vi "NI 5772 (AC) - Digitizer_vDirectDataSend (FPGA) V3.vi"() -> ()   [LabVIEW 2020]
doc: "Example Description:\nThis example demonstrates how to enable Time Interleaved Sampling with the NI 5772 adapter module to achieve a sampling rate of 1.6GS/s. This example continuously acquires records of analog input data from the NI 5772 adapter module. It allows you to select an AI channel, trigger type, and record size. This VI must be compiled before it is run. \n\nRunning the VI:\nThis VI must be run from the NI 5772 - Getting Started (Host).vi. Refer to the host VI documentation for steps regarding running and configuring the FPGA VI. \n\nExecution Steps:\nRefer to the Block Diagram of this VI for execution comments."
uses:
  Controls/AI Trigger Type.ctl
  Controls/DigitizerState.ctl
  Controls/Aquire State.ctl
  <vilib>/Platform/TimedLoop/XDataNode/timing_clust.ctl
  <vilib>/Platform/TimedLoop/XDataNode/nitl_modes.ctl
  <vilib>/Platform/TimedLoop/XDataNode/wakeup.ctl
  <vilib>/rvi/Emulation/niFpgaGetClockAttributes.vi
  <vilib>/rvi/Emulation/niFpgaSctlEmulationGetInTimedLoop.vi
  <vilib>/rvi/Emulation/niFpgaEmulationReportErrorSimple.vi
  <vilib>/rvi/eio/common/nirviEmuTemplateMethod_errors.vi
  <vilib>/rvi/Emulation/niFpgaCriticalErrorInLSC.vi
  <vilib>/rvi/Emulation/niFpgaProcessEmulError.vi
  <vilib>/rvi/Emulation/niFpgaEmulationIsFPGAContextNoSignature.vi
  <vilib>/rvi/errors/niFpgaSetErrorForExecOnDevCompSimple.vi
  <vilib>/rvi/eio/common/nirviEmuReportErrorAndStop.vi
  <vilib>/rvi/DataTransferAndStorage/Container/Common/niFpgaContainerGetUniqueNameForEmu.vi
  <vilib>/rvi/FIFO/Fifo_Resource/nirvififoEmulationSetSize.vi
  <vilib>/rvi/FIFO/Fifo_Resource/nirviFifoEmulationQueueMgr.vi
  <instcachedir>/0/nirviFifoEmulationQueueMgr_E5CAEC123FF24DC58D834DCA3CDAA9B5.lvgen/nirviFifoEmulationQueueMgr_E5CAEC123FF24DC58D834DCA3CDAA9B5_004.vi
  <vilib>/Utility/error.llb/Clear Errors.vi
  <vilib>/rvi/FIFO/Fifo_Resource/nirvififoEmulationCreateLock.vi
  <vilib>/rvi/FIFO/Fifo_Resource/nirvififoEmulationObtainLock.vi
  <vilib>/rvi/FIFO/Fifo_Resource/nirvififoEmulationReleaseLock.vi
  <vilib>/rvi/occurrence/nirviWaitOnOccurrenceBase.vi
  <vilib>/rvi/errors/nirviReportUnexpectedCaseInternalError.vi
  <vilib>/rvi/errors/nirviReportUnexpectedCaseInternalError (U32).vi
  <vilib>/rvi/FIFO/Fifo_Resource/nirvififoEmulationDetermineInputValidOut.vi
  <instcachedir>/0/nirviFifoEmulationQueueMgr_E5CAEC123FF24DC58D834DCA3CDAA9B5.lvgen/nirviFifoEmulationQueueMgr_E5CAEC123FF24DC58D834DCA3CDAA9B5_000.vi
  <instrlib>/_niInstr/Basic Elements/v1/FPGA/Private/Count Up U64.vi
  <instcachedir>/0/nirviFifoEmulationQueueMgr_E5CAEC123FF24DC58D834DCA3CDAA9B5.lvgen/nirviFifoEmulationQueueMgr_E5CAEC123FF24DC58D834DCA3CDAA9B5_003.vi
  <vilib>/rvi/interface/RandomDataEmulation/niFpgaRandomDataHandleErrors.vi
  <vilib>/eio/EIONode/EIONode.xnode
  <vilib>/rvi/DataTransferAndStorage/Container/XNode/niFpgaContainer.xnode
  <vilib>/rvi/FIFO/Fifo_Resource/nirvififoEmulationRead.vi
  <vilib>/Platform/TimedLoop/XDataNode/XDataNode.xnode
  <vilib>/rvi/FIFO/Fifo_Resource/nirvififoEmulationWrite.vi
  <vilib>/rvi/FIFO/Fifo_Resource/nirvififoEmulationGetNumberOfElementsToRead.vi
  <vilib>/rvi/interface/RandomDataEmulation/nirviRandomDataFpgaReadWriteTemplate.vi
  <vilib>/Platform/TimedLoop/XDataNode/XDNodeRunTimeDep.lvlib
  <instrlib>/_niInstr/Basic Elements/v1/FPGA/niInstr Basic Elements v1 FPGA.lvlib
  <vilib>/rvi/Memory/Memory_Emulation/nirvimemoryFastEmulation.vi
  <vilib>/rvi/Memory/Memory_Emulation/nirvimemoryEmulation.vi
panel:
  out "Accumulator Length":u32
  out "Aquire Loop":T1
  out "Data Transfer Loop":T2
  out "DMA FIFO Overflow? 3":bool caption="FIFO Overflow?"
  out "DMA FIFO Overflow? 2":bool caption="FIFO Overflow?"
  out "WaitForWave\nCompletion":u16
  in  "Wave Sampling Rate":sgl
  in  "WaveSampleCount":sgl format="%#_13g"
  in  "Delay (us)":sgl
  in  "AvgCount_powerOf2":i16=1
  out "DMA FIFO Overflow?":bool caption="FIFO Overflow?"
  out "Removed\nElement":u64
  out "AvgCount":u16=1
  in  "vi/nGenTrig":bool
  in  "TrigIn Simulate":bool
  out "Trig Count":u64
  in  "Clear Count":bool
  out "Delay after Trig [cycles]":u16
  out "TS FIFO In Overflow?":bool caption="FIFO Overflow?"
  in  "Samples Per Trigger":u16=512 min=1 step=1
  in  "Arm Trigger":bool
  in  "User Command Commit":bool
  in  "User Command":u8
  out "User Command Idle":bool
  out "User Command Status":u8
  in  "User Data 0":u16
  in  "User Data 1":u8
  out "PLL Locked":bool
  out "User Error":bool
  out "Configured?":bool
  in  "Trigger Level":i16
  in  "Trigger Type":T3
  # "Resource Configuration"
  # "Analog Input"
  # "Clock Configuration"
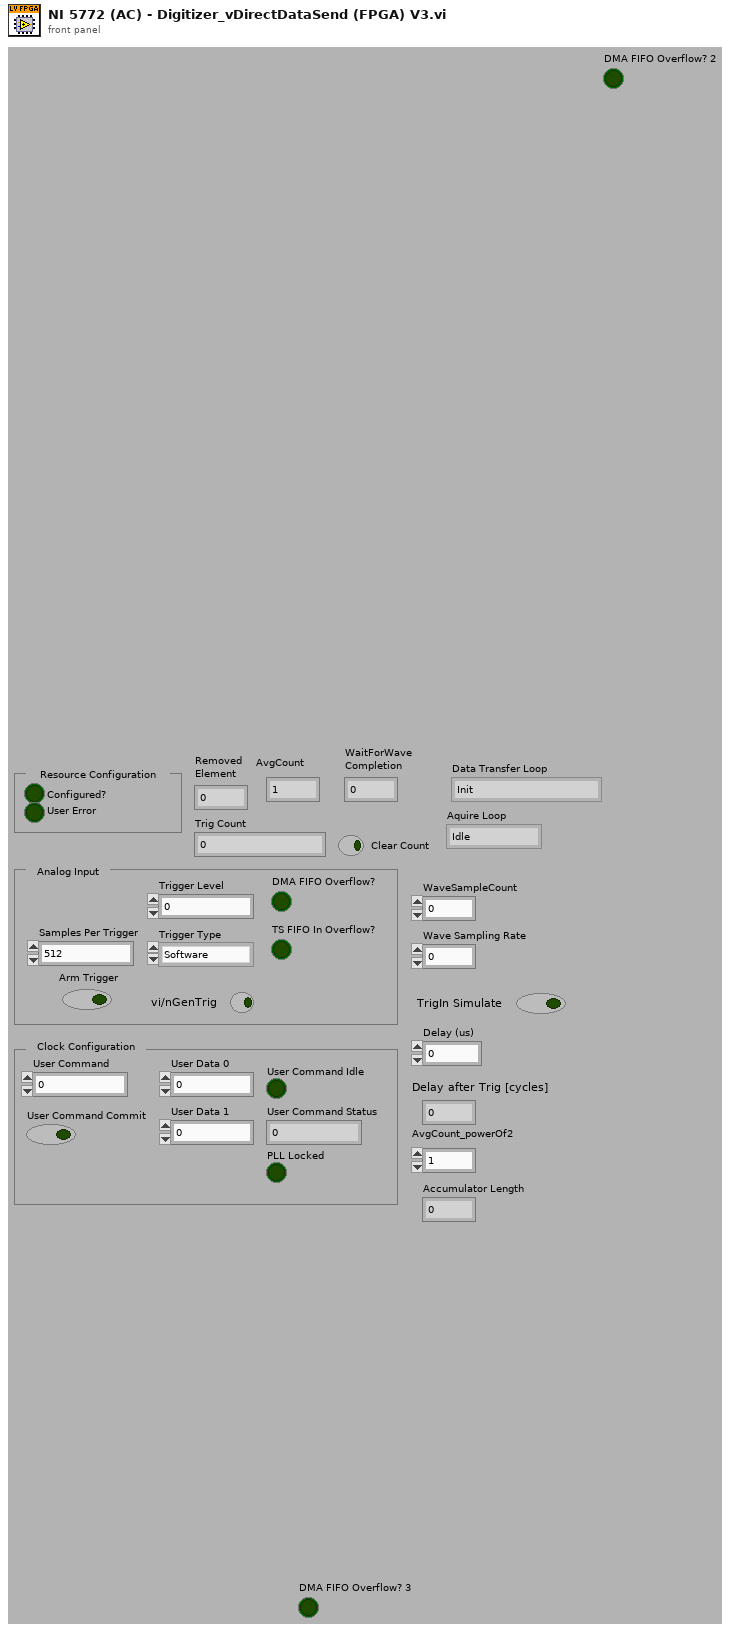
[diagram p1: front panel]
types:
  T1 = typedef "Aquire State.ctl" = enum8{"Idle", "Wait for Trigger", "AlignWave", "Hold Aquire", "Acquire", "WaitForWaveCompletion", "CheckAvg"}
  T2 = typedef "DigitizerState.ctl" = enum16{"Init", "Build/Clear Accumulator", "GetData", "AverageCountCheck", "SendtoHost"}
  T3 = typedef "AI Trigger Type.ctl" = enum8{"Software", "Data Edge"}
  T4 = typedef "XDNodeRunTimeDep.lvlib/timing_clust.ctl" = cluster{"Expected End [f-1]":u64, "Actual End [f-1]":u64, "Finished Late? [f-1]":bool, "Expected End [i-1]":u64, "Actual End [i-1]":u64, "Finished Late? [i-1]":bool, "Expected Start [i]":u64, "Actual Start [i]":u64, "Expected Start [f]":u64, "Actual Start [f]":u64, "Source Name":string, "Structure Name":string, "Period":i64, "Deadline":i64, "Offset":i64, "Start":i64, "Priority":i32, "Timeout":i32, "Mode":T5, "Wakeup Reason":T6, "Error":errorcluster, "Source Type":string, "Secondary Source Type":string, "Global End Time":u64, "Global Start Time":u64, "Frame Duration":u64, "Iteration Duration":u64, "Assigned CPU":i32, "I/O Scan Engine Mode":u32}
  T5 = typedef "XDNodeRunTimeDep.lvlib/nitl_modes.ctl" = enum32{"No Change", "Process missed periods, maintain original phase", "Discard missed periods, maintain original phase", "Process missed periods, ignore original phase", "Discard missed periods, ignore original phase"}
  T6 = typedef "XDNodeRunTimeDep.lvlib/wakeup.ctl" = enum32{"Normal", "Aborted", "Asynchronous wakeup", "Timing source error", "Timed loop error", "Timeout"}
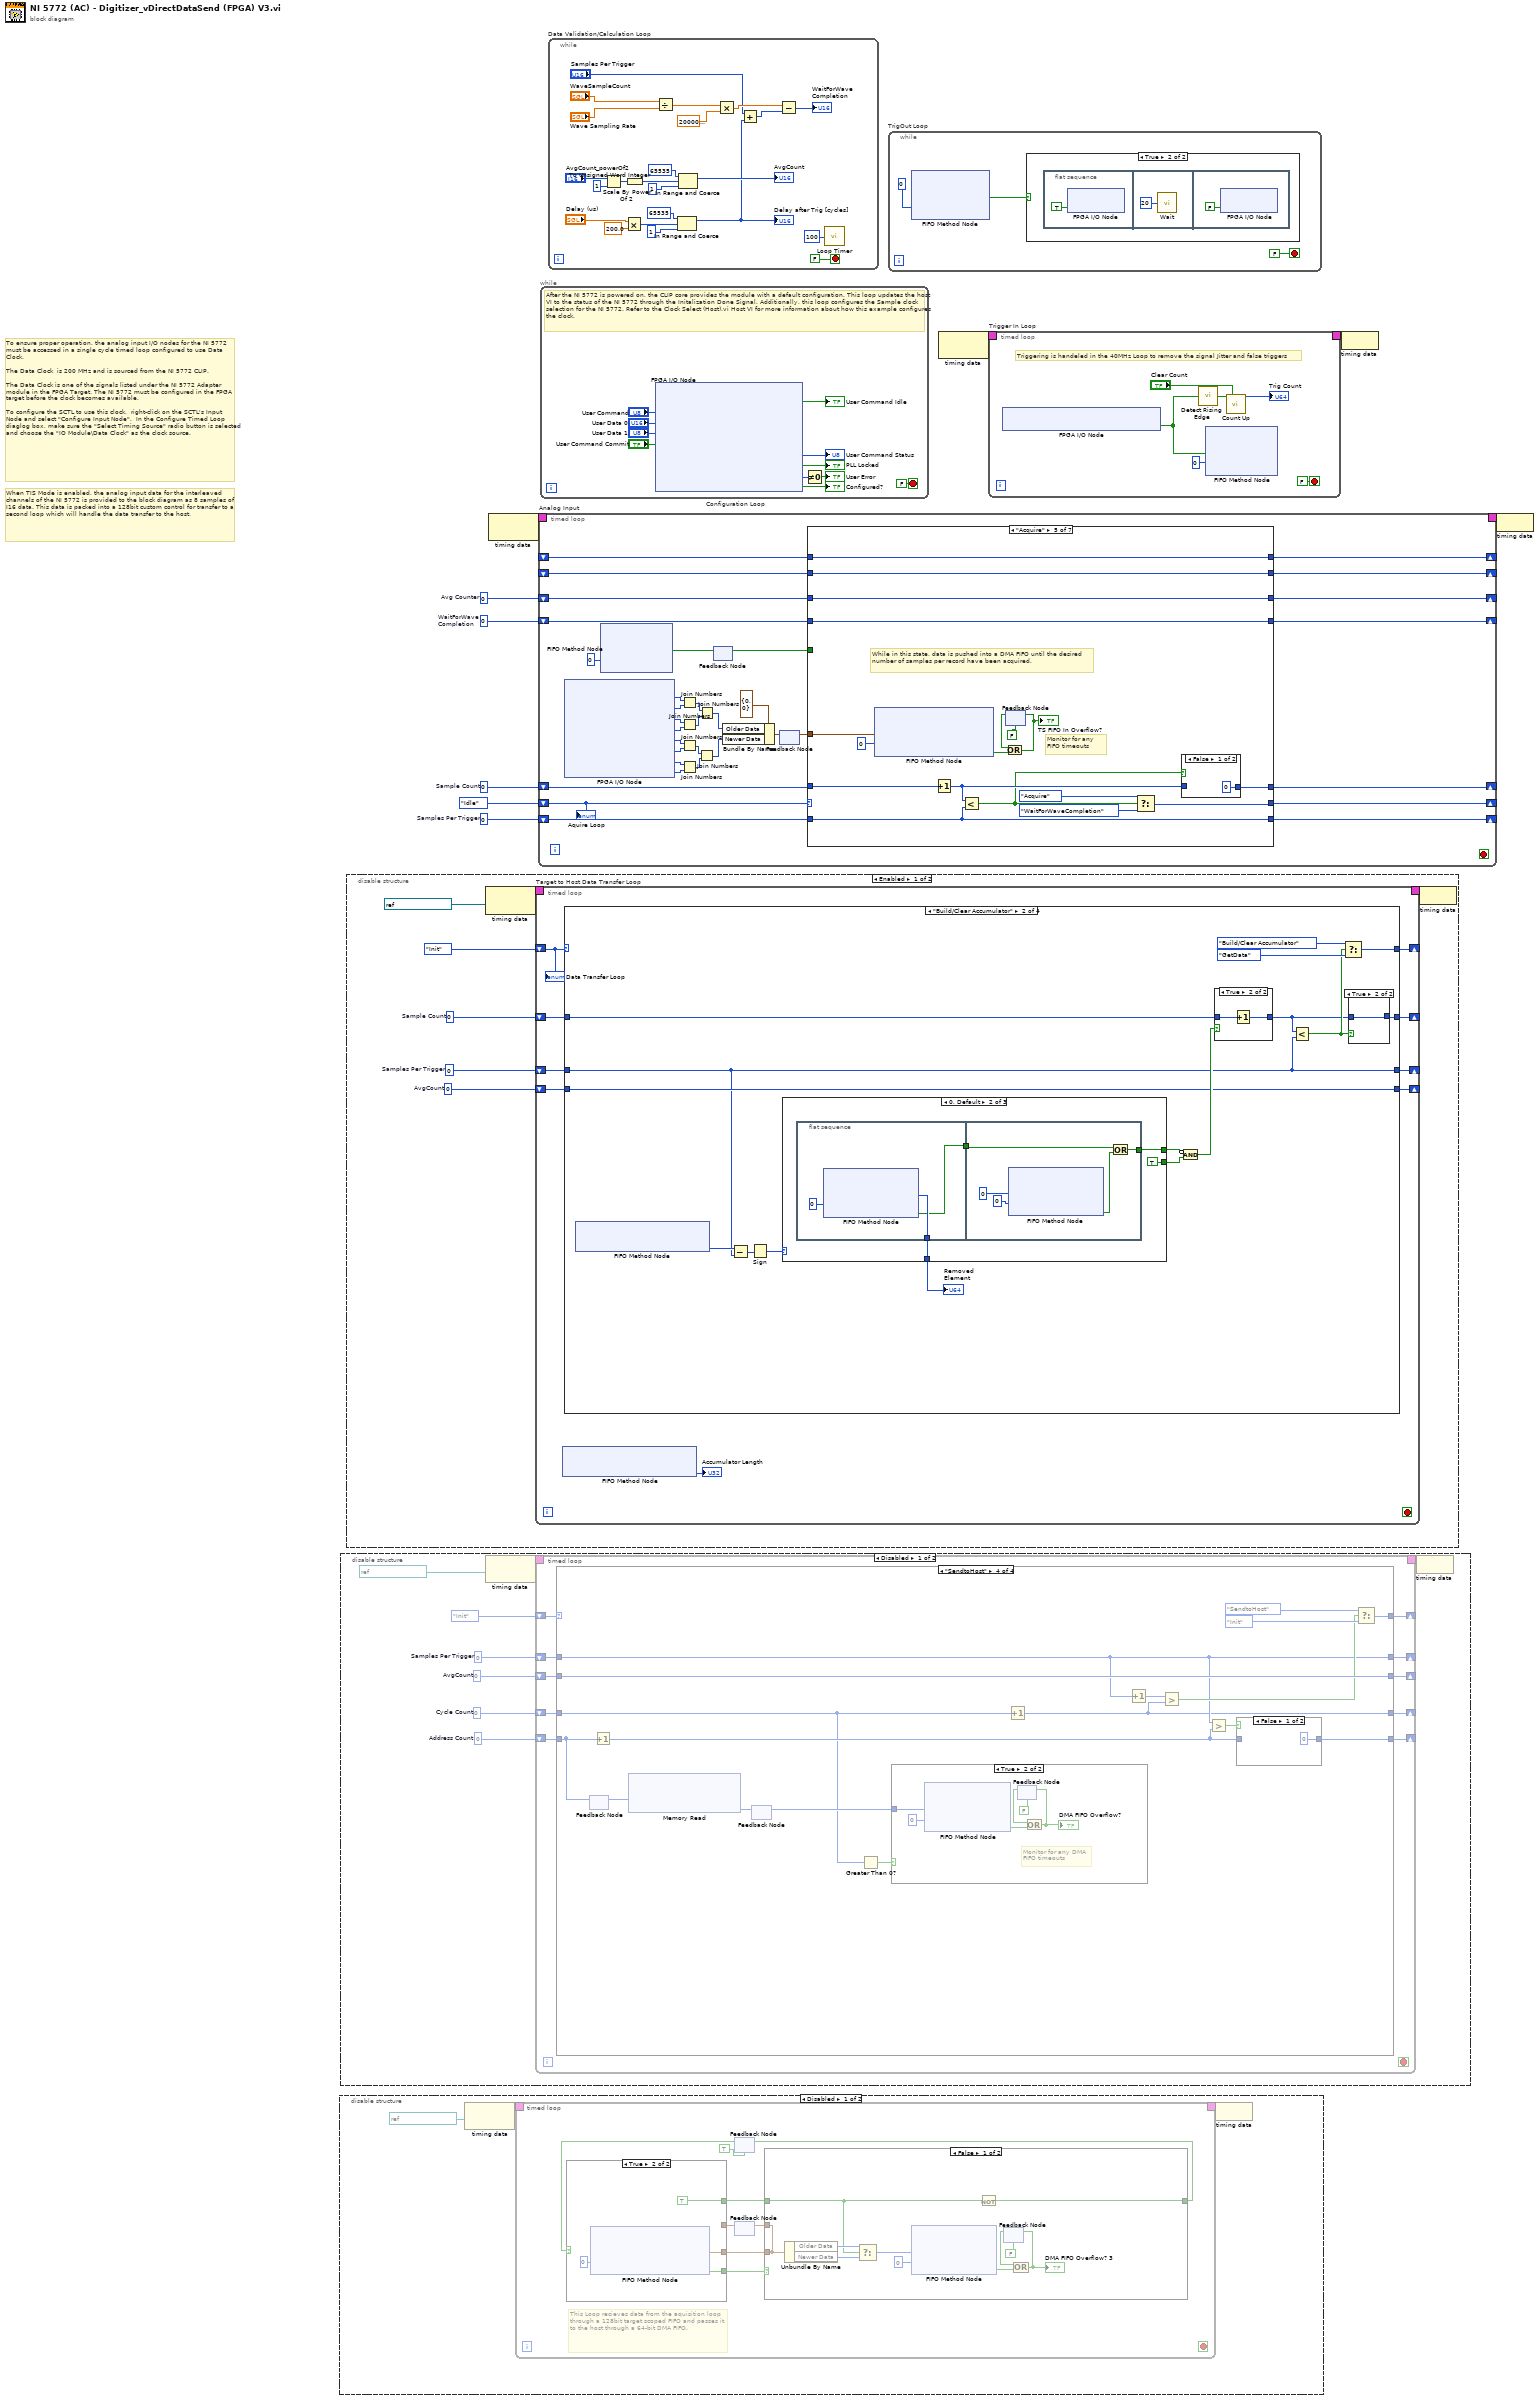
[diagram p0: block diagram]
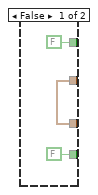
[diagram p2: hidden frame]
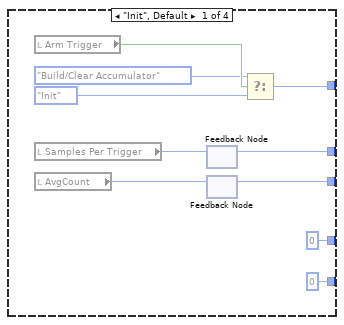
[diagram p5: hidden frame]
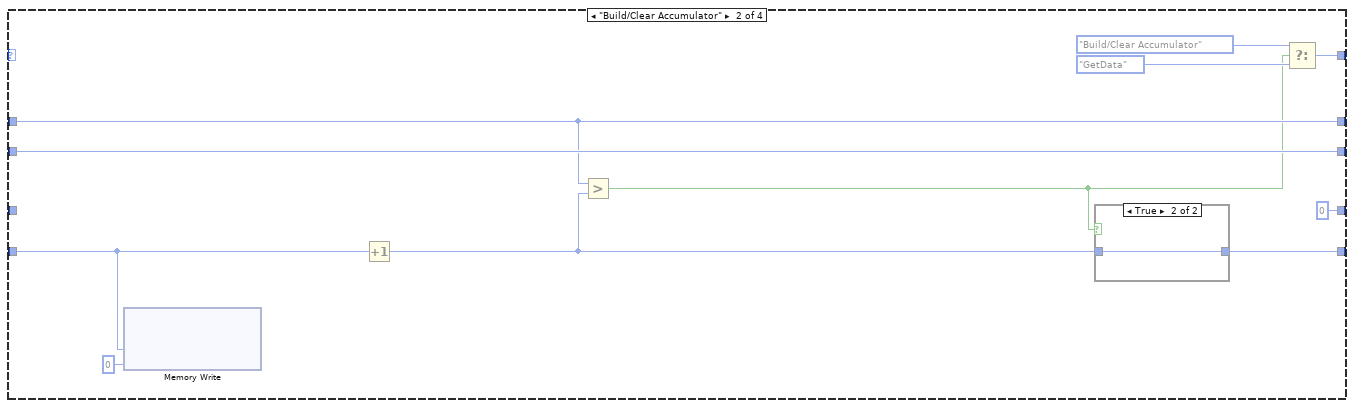
[diagram p6: hidden frame]
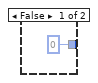
[diagram p7: hidden frame]
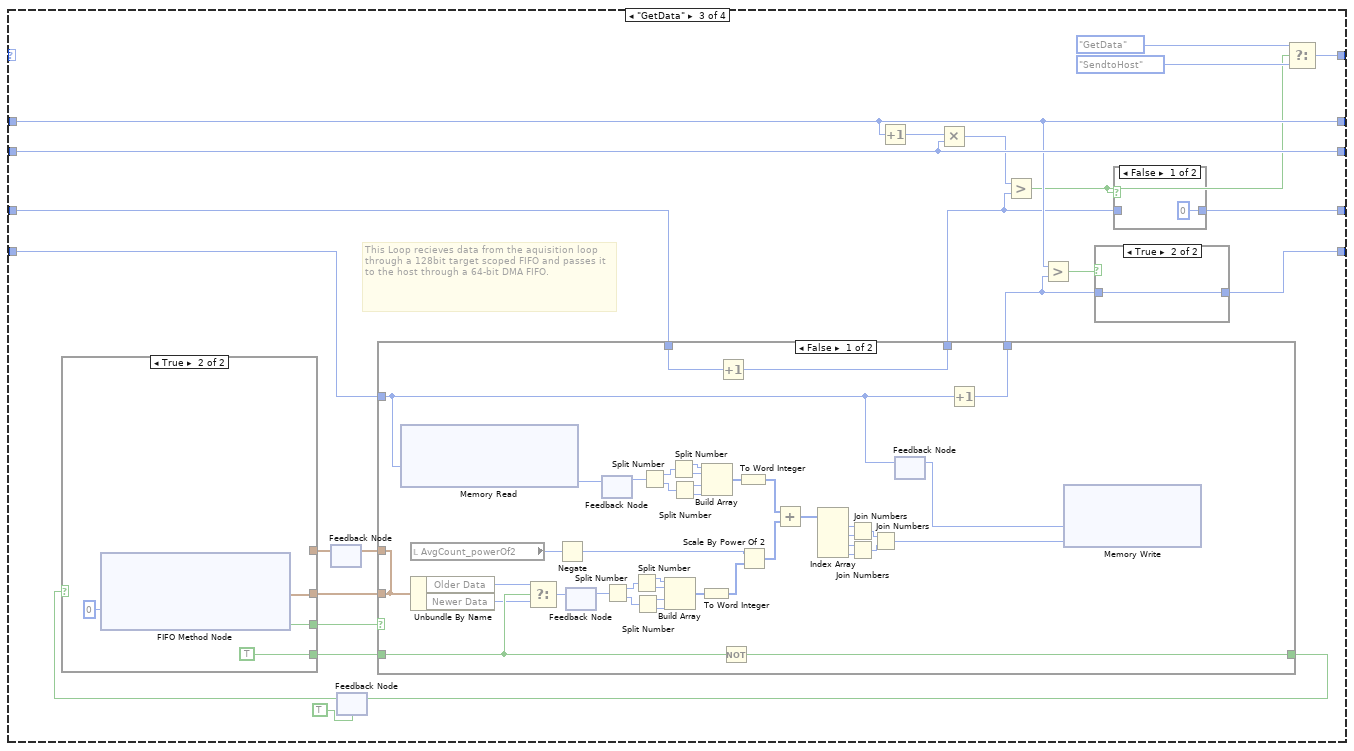
[diagram p8: hidden frame]
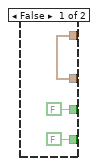
[diagram p10: hidden frame]
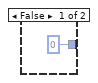
[diagram p12: hidden frame]
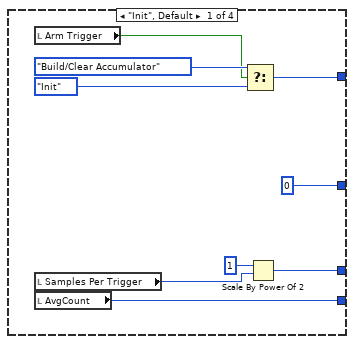
[diagram p16: hidden frame]
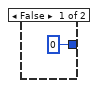
[diagram p17: hidden frame]
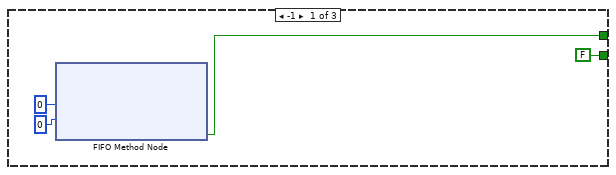
[diagram p19: hidden frame]
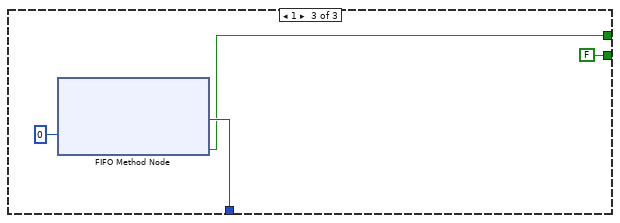
[diagram p20: hidden frame]
diagram:
  w1 = u16 0  # WaitForWave Completion
  w2 = u16 0  # Avg Counter
  w5 = u16 0  # Samples Per Trigger
  w6 = u16 0  # Sample Count
  # "When TIS Mode is enabled, the analog input data for the interleaved channels of the NI 5772 is provided to the block diagram as 8 samples of I16 data. This data is packed into a 128bit custom control for transfer to a second loop which will handle the data transfer to the host."
  # "To ensure proper operation, the analog input I/O nodes for the NI 5772 must be accessed in a single cycle timed loop configured to use Data Clock. \n\nThe Data Clock  is 200 MHz and is sourced from the NI 5772 CLIP.\n\nThe Data Clock is one of the signals listed under the NI 5772 Adapter module in the FPGA Target. The NI 5772 must be configured in the FPGA target before the clock becomes available. \n\nTo configure the SCTL to use this clock,  right-click on the SCTL's Input Node and select \"Configure Input Node\".  In the Configure Timed Loop diaglog box, make sure the \"Select Timing Source\" radio button is selected and choose the \"IO Module\\Data Clock\" as the clock source."
  n1 = disable-structure shown="Disabled" {
    frame Disabled {
      n2 = node-c288(refnum<k21> "100 MHz Clock" ("Source Name")) -> (w12:T4)
      n3 = timed-loop {
        timing: w12 -> [_]
        timing-out: [_] -> w11
        stop <- _ stop-if-true
        # "This Loop recieves data from the aquisition loop through a 128bit target scoped FIFO and passes it to the host through a 64-bit DMA FIFO."
        n4 = feedback #1(TRUE ("Timed Out?")) -> (w15:bool)
        n5 = feedback #2() -> (w16:cluster{"Older Data":u64, "Newer Data":u64})  [unwired: 1 in]
        n6 = case shown="True" w15 {
          tunnel: [w21 w24] -> w18
          tunnel: [FALSE ("Timed Out?") w25] -> w20
          tunnel: [FALSE ("Timed Out?") TRUE ("Timed Out?")] -> w19
          tunnel: w16 -> [w21 _]
          frame False {
          }
          frame True {
            n7 = xnode ("FIFO Method Node")("Timeout"=0) -> ("Element"=w24:cluster{"Older Data":u64, "Newer Data":u64}, "Timed Out?"=w25:bool)  [unwired: 1 in, 1 out]
          }
        }
        n8 = case shown="False" w20 {
          tunnel: [w36 w40] -> w14
          tunnel: w19 -> [w37 w40]
          tunnel: w18 -> [w35 w39]
          tunnel: [w35 w39] -> w17
          frame False {
            n9 = Unbundle By Name(w35) -> ("Older Data"=w38:u64, "Newer Data"=w34:u64)
            n10 = Select(t=w38, s=w37, f=w34) -> (s? t:f=w28:u64)
            n11 = xnode ("FIFO Method Node")("Element"=w28, "Timeout"=0) -> ("Timed Out?"=w30:bool)  [unwired: 1 in, 1 out]
            n12 = Not(x=w37) -> (.not. x?=w36:bool)
            n13 = feedback #3(FALSE) -> (w31:bool)
            n14 = Compound Arithmetic op=OR(w31, w30) -> (w29:bool)
            "DMA FIFO Overflow? 3" <- w29
            n15 = feedback-in #3(w29) -> ()
          }
          frame True {
          }
        }
        n16 = feedback-in #1(w14) -> ()
        n17 = feedback-in #2(w17) -> ()
      }
      n18 = node-c288(w11) -> ()
    }
    frame Enabled {
    }
  }
  n19 = disable-structure shown="Disabled" {
    frame Disabled {
      w47 = u32 0  # Cycle Count
      w48 = u32 0  # Address Count
      w49 = u16 0  # AvgCount
      w50 = u16 0  # Samples Per Trigger
      n20 = node-c288(refnum<k21> "100 MHz Clock" ("Source Name")) -> (w54:T4)
      n21 = timed-loop {
        timing: w54 -> [_]
        timing-out: [_] -> w53
        shift-right: [w63] -> _
        shift-left: DigitizerState."Init" -> [w64]
        shift-right: [w62] -> _
        shift-left: w50 -> [w60]
        shift-right: [w61] -> _
        shift-left: w49 -> [w59]
        shift-right: [w57] -> _
        shift-left: w48 -> [w58]
        shift-right: [w55] -> _
        shift-left: w47 -> [w56]
        stop <- _ stop-if-true
        n22 = case shown="\"SendtoHost\"" w64 {
          tunnel: [w69 w79 w108 w180] -> w63
          tunnel: [w68 w82 w92 w170] -> w62
          tunnel: [w67 w83 w98 w183] -> w61
          tunnel: w60 -> [_ w82 w92 w170]
          tunnel: w59 -> [_ w83 w98 w183]
          tunnel: w58 -> [_ w85 w95 w172]
          tunnel: [u32 0 w76 w107 w178] -> w57
          tunnel: w56 -> [_ _ w91 w167]
          tunnel: [u32 0 ("Cycle Count") u32 0 ("Cycle Count") w88 w168] -> w55
          frame "Init", Default {
            n23 = local read "Arm Trigger"() -> (w74:bool)
            n24 = local read "Samples Per Trigger"() -> (w70:u16)
            n25 = local read "AvgCount"() -> (w71:u16)
            n26 = feedback #4() -> (w68:u16)  [unwired: 1 in]
            n27 = feedback-in #4(w70) -> ()
            n28 = feedback #5() -> (w67:u16)  [unwired: 1 in]
            n29 = feedback-in #5(w71) -> ()
            n30 = Select(t=DigitizerState."Build/Clear Accumulator", s=w74, f=DigitizerState."Init") -> (s? t:f=w69:T2)
          }
          frame "Build/Clear Accumulator" {
            n31 = xnode ("Memory Write")("Address"=w85, "Data"=u64 0) -> ()  [unwired: 1 in, 1 out]
            n32 = Increment(x=w85) -> (x+1=w77:u32)
            n33 = Greater?(x=w82, y=w77) -> (0:w78:bool)
            n34 = case shown="True" w78 {
              tunnel: w77 -> [_ w87]
              tunnel: [u32 0 w87] -> w76
              frame False {
              }
              frame True {
              }
            }
            n35 = Select(t=DigitizerState."Build/Clear Accumulator", s=w78, f=DigitizerState."GetData") -> (s? t:f=w79:T2)
          }
          frame "GetData" {
            # "This Loop recieves data from the aquisition loop through a 128bit target scoped FIFO and passes it to the host through a 64-bit DMA FIFO."
            n36 = feedback #6() -> (w102:cluster{"Older Data":u64, "Newer Data":u64})  [unwired: 1 in]
            n37 = feedback #7(TRUE ("Timed Out?")) -> (w101:bool)
            n38 = case shown="True" w101 {
              tunnel: [w113 w116] -> w104
              tunnel: [FALSE ("Timed Out?") w117] -> w106
              tunnel: [FALSE ("Timed Out?") TRUE ("Timed Out?")] -> w105
              tunnel: w102 -> [w113 _]
              frame False {
              }
              frame True {
                n39 = xnode ("FIFO Method Node")("Timeout"=0) -> ("Element"=w116:cluster{"Older Data":u64, "Newer Data":u64}, "Timed Out?"=w117:bool)  [unwired: 1 in, 1 out]
              }
            }
            n40 = case shown="False" w106 {
              tunnel: [w158 w164] -> w100
              tunnel: w105 -> [w159 w164]
              tunnel: w104 -> [w157 w163]
              tunnel: [w157 w163] -> w103
              tunnel: w95 -> [w134 w162]
              tunnel: [w147 w162] -> w94
              tunnel: w91 -> [w123 w161]
              tunnel: [w122 w161] -> w89
              frame False {
                n41 = xnode ("Memory Read")("Address"=w134) -> ("Data"=w125:u64)  [unwired: 1 in, 1 out]
                n42 = local read "AvgCount_powerOf2"() -> (w138:i16)
                n43 = Unbundle By Name(w157) -> ("Older Data"=w160:u64, "Newer Data"=w156:u64)
                n44 = Select(t=w160, s=w159, f=w156) -> (s? t:f=w148:u64)
                n45 = Negate(x=w138) -> (-x=w139:i16)
                n46 = feedback-in #8(w148) -> ()
                n47 = feedback #8() -> (w121:u64)  [unwired: 1 in]
                n48 = feedback-in #9(w125) -> ()
                n49 = feedback #9() -> (w124:u64)  [unwired: 1 in]
                n50 = Split Number(x=w121) -> (hi(x)=w150:u32, lo(x)=w151:u32)
                n51 = Split Number(x=w150) -> (hi(x)=w152:u16, lo(x)=w153:u16)
                n52 = Split Number(x=w151) -> (hi(x)=w154:u16, lo(x)=w155:u16)
                n53 = Split Number(x=w124) -> (hi(x)=w146:u32, lo(x)=w145:u32)
                n54 = Build Array(w152, w153, w154, w155) -> (w149:u16[])
                n55 = Split Number(x=w146) -> (hi(x)=w144:u16, lo(x)=w143:u16)
                n56 = Split Number(x=w145) -> (hi(x)=w142:u16, lo(x)=w141:u16)
                n57 = To Word Integer(number=w149) -> (16bit integer=w137:i16[])
                n58 = Build Array(w144, w143, w142, w141) -> (w140:u16[])
                n59 = Increment(x=w123) -> (x+1=w122:u32)
                n60 = Not(x=w159) -> (.not. x?=w158:bool)
                n61 = To Word Integer(number=w140) -> (16bit integer=w135:i16[])
                n62 = Scale By Power Of 2(n=w139, x=w137) -> (x*2^n=w136:i16[])
                n63 = Add(x=w135, y=w136) -> (x+y=w127:i16[])
                n64 = Index Array(array=w127) -> (element #1=w130:i16, element #2=w131:i16, element #3=w132:i16, element #4=w133:i16)  [unwired: 4 in]
                n65 = Join Numbers(hi=w130, lo=w131) -> ((hi.lo)=w128:u32)
                n66 = Join Numbers(hi=w132, lo=w133) -> ((hi.lo)=w129:u32)
                n67 = Join Numbers(hi=w128, lo=w129) -> ((hi.lo)=w126:u64)
                n68 = feedback-in #10(w134) -> ()
                n69 = feedback #10() -> (w120:u32)  [unwired: 1 in]
                n70 = Increment(x=w134) -> (x+1=w147:u32)
                n71 = xnode ("Memory Write")("Address"=w120, "Data"=w126) -> ()  [unwired: 1 in, 1 out]
              }
              frame True {
              }
            }
            n72 = feedback-in #6(w103) -> ()
            n73 = feedback-in #7(w100) -> ()
            n74 = Increment(x=w92) -> (x+1=w93:u16)
            n75 = Multiply(x=w93, y=w98) -> (x*y=w97:u16)
            n76 = Greater?(x=w97, y=w89) -> (0:w90:bool)
            n77 = Greater?(x=w92, y=w94) -> (0:w96:bool)
            n78 = case shown="True" w96 {
              tunnel: w94 -> [_ w166]
              tunnel: [u32 0 w166] -> w107
              frame False {
              }
              frame True {
              }
            }
            n79 = case shown="False" w90 {
              tunnel: w89 -> [_ w112]
              tunnel: [u32 0 ("Cycle Count") w112] -> w88
              frame False {
              }
              frame True {
              }
            }
            n80 = Select(t=DigitizerState."GetData", s=w90, f=DigitizerState."SendtoHost") -> (s? t:f=w108:T2)
          }
          frame "SendtoHost" {
            n81 = feedback-in #11(w172) -> ()
            n82 = feedback #11() -> (w174:u32)  [unwired: 1 in]
            n83 = Increment(x=w172) -> (x+1=w169:u32)
            n84 = xnode ("Memory Read")("Address"=w174) -> ("Data"=w177:u64)  [unwired: 1 in, 1 out]
            n85 = feedback-in #12(w177) -> ()
            n86 = feedback #12() -> (w176:u64)  [unwired: 1 in]
            n87 = Greater Than 0?(x=w167) -> (x > 0?=w173:bool)
            n88 = case shown="True" w173 {
              tunnel: w176 -> [_ w184]
              frame False {
              }
              frame True {
                # "Monitor for any DMA FIFO timeouts"
                n89 = xnode ("FIFO Method Node")("Element"=w184, "Timeout"=0) -> ("Timed Out?"=w188:bool)  [unwired: 1 in, 1 out]
                n90 = feedback #13(FALSE) -> (w187:bool)
                n91 = Compound Arithmetic op=OR(w187, w188) -> (w189:bool)
                "DMA FIFO Overflow?" <- w189
                n92 = feedback-in #13(w189) -> ()
              }
            }
            n93 = Increment(x=w167) -> (x+1=w168:u32)
            n94 = Increment(x=w170) -> (x+1=w175:u16)
            n95 = Greater?(x=w175, y=w168) -> (0:w179:bool)
            n96 = Greater?(x=w170, y=w169) -> (0:w171:bool)
            n97 = case shown="False" w171 {
              tunnel: w169 -> [_ w191]
              tunnel: [u32 0 w191] -> w178
              frame False {
              }
              frame True {
              }
            }
            n98 = Select(t=DigitizerState."SendtoHost", s=w179, f=DigitizerState."Init") -> (s? t:f=w180:T2)
          }
        }
      }
      n99 = node-c288(w53) -> ()
    }
    frame Enabled {
    }
  }
  n100 = disable-structure shown="Enabled" {
    frame Enabled {
      w198 = u16 0  # Sample Count
      w199 = u16 0  # Samples Per Trigger
      w200 = u16 0  # AvgCount
      n101 = node-c288(refnum<k21> "100 MHz Clock" ("Source Name")) -> (w204:T4)
      n102 = timed-loop "Target to Host Data Transfer Loop" {
        timing: w204 -> [_]
        timing-out: [_] -> w203
        shift-right: [w208] -> _
        shift-left: DigitizerState."Init" -> [w213]
        shift-right: [w212] -> _
        shift-left: w199 -> [w211]
        shift-right: [w210] -> _
        shift-left: w200 -> [w209]
        shift-right: [w206] -> _
        shift-left: w198 -> [w207]
        stop <- _ stop-if-true
        n103 = xnode ("FIFO Method Node")() -> ("Number of Elements to Read"=→"Accumulator Length":u32)  [unwired: 1 in, 1 out]
        n104 = case shown="\"Build/Clear Accumulator\"" w213 {
          tunnel: [w215 w226 w274 w348] -> w212
          tunnel: w211 -> [_ w226 w274 w348]
          tunnel: [w222 w227 w273 w355] -> w210
          tunnel: w209 -> [_ w227 w273 w355]
          tunnel: [w218 w234 w268 w351] -> w208
          tunnel: w207 -> [_ w229 w267 w349]
          tunnel: [u16 0 ("Sample Count") w223 w266 w346] -> w206
          frame "Init", Default {
            n105 = local read "Arm Trigger"() -> (w219:bool)
            n106 = local read "Samples Per Trigger"() -> (w214:u16)
            n107 = local read "AvgCount"() -> (w222:u16)
            n108 = Select(t=DigitizerState."Build/Clear Accumulator", s=w219, f=DigitizerState."Init") -> (s? t:f=w218:T2)
            n109 = Scale By Power Of 2(n=i16 1, x=w214) -> (x*2^n=w215:u16)
          }
          frame "Build/Clear Accumulator" {
            n110 = xnode ("FIFO Method Node")() -> ("Number of Elements to Read"=w238:u32)  [unwired: 1 in, 1 out]
            n111 = Subtract(x=w238, y=w226) -> (x-y=w237:i8)
            n112 = Sign(1:w237) -> (0:w236:i8)
            n113 = case shown="0, Default" w236 {
              tunnel: [_ w251 w262] -> w235
              tunnel: [w245 w249 w261] -> w231
              tunnel: [FALSE TRUE FALSE] -> w230
              frame -1 {
                n114 = xnode ("FIFO Method Node")("Element"=u64 0, "Timeout"=0) -> ("Timed Out?"=w245:bool)  [unwired: 1 in, 1 out]
              }
              frame 0, Default {
                n115 = flat-sequence {
                  tunnel: [w253] -> w251
                  tunnel: [w252] -> w250
                  tunnel: w250 -> [w257]
                  tunnel: [w255] -> w249
                  frame #0 {
                    n116 = xnode ("FIFO Method Node")("Timeout"=0) -> ("Element"=w253:u64, "Timed Out?"=w252:bool)  [unwired: 1 in, 1 out]
                  }
                  frame #1 {
                    n117 = xnode ("FIFO Method Node")("Element"=u64 0 ("y"), "Timeout"=0) -> ("Timed Out?"=w256:bool)  [unwired: 1 in, 1 out]
                    n118 = Compound Arithmetic op=OR(w257, w256) -> (w255:bool)
                  }
                }
              }
              frame 1 {
                n119 = xnode ("FIFO Method Node")("Timeout"=0) -> ("Element"=w262:u64, "Timed Out?"=w261:bool)  [unwired: 1 in, 1 out]
              }
            }
            "Removed\nElement" <- w235
            n120 = Compound Arithmetic op=AND(invert w231, w230) -> (w228:bool)
            n121 = case shown="True" w228 {
              tunnel: w229 -> [w241 w243]
              tunnel: [w241 w242] -> w224
              frame False {
              }
              frame True {
                n122 = Increment(x=w243) -> (x+1=w242:u16)
              }
            }
            n123 = Less?(x=w224, y=w226) -> (x < y?=w225:bool)
            n124 = Select(t=DigitizerState."Build/Clear Accumulator", s=w225, f=DigitizerState."GetData") -> (s? t:f=w234:T2)
            n125 = case shown="True" w225 {
              tunnel: [u16 0 ("Sample Count") w240] -> w223
              tunnel: w224 -> [_ w240]
              frame False {
              }
              frame True {
              }
            }
          }
          frame "GetData" {
            # "This Loop recieves data from the aquisition loop through a 128bit target scoped FIFO and passes it to the host through a 64-bit DMA FIFO."
            n126 = Multiply(x=w274, y=w273) -> (x*y=w265:u16)
            n127 = feedback #14(TRUE ("Timed Out?")) -> (w279:bool)
            n128 = feedback #15() -> (w278:cluster{"Older Data":u64, "Newer Data":u64})  [unwired: 1 in]
            n129 = case shown="True" w279 {
              tunnel: [w287 w290] -> w276
              tunnel: [FALSE ("Timed Out?") w291] -> w264
              tunnel: [FALSE ("Timed Out?") TRUE ("Timed Out?")] -> w275
              tunnel: w278 -> [w287 _]
              frame False {
              }
              frame True {
                n130 = xnode ("FIFO Method Node")("Timeout"=0) -> ("Element"=w290:cluster{"Older Data":u64, "Newer Data":u64}, "Timed Out?"=w291:bool)  [unwired: 1 in, 1 out]
              }
            }
            n131 = case shown="False" w264 {
              tunnel: [w308 w344] -> w280
              tunnel: w275 -> [w309 w344]
              tunnel: w276 -> [w307 w343]
              tunnel: [w307 w343] -> w277
              tunnel: [w295 FALSE ("increment")] -> _
              frame False {
                n132 = flat-sequence {
                  tunnel: [w311] -> w299
                  tunnel: [w322] -> w297
                  tunnel: w294 -> [w318]
                  tunnel: w299 -> [w337]
                  tunnel: [w334] -> w295
                  tunnel: w297 -> [w336]
                  frame #0 {
                    n133 = xnode ("FIFO Method Node")("Timeout"=0) -> ("Element"=w321:u64, "Timed Out?"=w322:bool)  [unwired: 1 in, 1 out]
                    n134 = local read "AvgCount_powerOf2"() -> (w320:i16)
                    n135 = Negate(x=w320) -> (-x=w319:i16)
                    n136 = Split Number(x=w321) -> (hi(x)=w327:u32, lo(x)=w328:u32)
                    n137 = Split Number(x=w327) -> (hi(x)=w329:u16, lo(x)=w330:u16)
                    n138 = Split Number(x=w328) -> (hi(x)=w331:u16, lo(x)=w332:u16)
                    n139 = Build Array(w329, w330, w331, w332) -> (w333:u16[])
                    n140 = To Word Integer(number=w333) -> (16bit integer=w325:i16[])
                    n141 = Scale By Power Of 2(n=w319, x=w318) -> (x*2^n=w317:i16[])
                    n142 = Add(x=w317, y=w325) -> (x+y=w316:i16[])
                    n143 = Index Array(array=w316) -> (element #1=w315:i16, element #2=w314:i16, element #3=w313:i16, element #4=w312:i16)  [unwired: 4 in]
                    n144 = Join Numbers(hi=w315, lo=w314) -> ((hi.lo)=w324:u32)
                    n145 = Join Numbers(hi=w313, lo=w312) -> ((hi.lo)=w323:u32)
                    n146 = Join Numbers(hi=w324, lo=w323) -> ((hi.lo)=w311:u64)
                  }
                  frame #1 {
                    n147 = case shown="False" w336 {
                      tunnel: w337 -> [w339 _]
                      tunnel: [w338 TRUE ("Timed Out?")] -> w335
                      frame False {
                        n148 = xnode ("FIFO Method Node")("Element"=w339, "Timeout"=0) -> ("Timed Out?"=w338:bool)  [unwired: 1 in, 1 out]
                      }
                      frame True {
                      }
                    }
                    n149 = Not(x=w335) -> (.not. x?=w334:bool)
                  }
                }
                n150 = Unbundle By Name(w307) -> ("Older Data"=w310:u64, "Newer Data"=w306:u64)
                n151 = Select(t=w310, s=w309, f=w306) -> (s? t:f=w296:u64)
                n152 = Split Number(x=w296) -> (hi(x)=w300:u32, lo(x)=w301:u32)
                n153 = Split Number(x=w300) -> (hi(x)=w302:u16, lo(x)=w303:u16)
                n154 = Split Number(x=w301) -> (hi(x)=w304:u16, lo(x)=w305:u16)
                n155 = Build Array(w302, w303, w304, w305) -> (w298:u16[])
                n156 = To Word Integer(number=w298) -> (16bit integer=w294:i16[])
                n157 = Not(x=w309) -> (.not. x?=w308:bool)
              }
              frame True {
              }
            }
            n158 = feedback-in #14(w280) -> ()
            n159 = feedback-in #15(w277) -> ()
            n160 = case shown="False" w264 {
              tunnel: w267 -> [w285 w286]
              tunnel: [w284 w286] -> w269
              frame False {
                n161 = Increment(x=w285) -> (x+1=w284:u16)
              }
              frame True {
              }
            }
            n162 = Less?(x=w269, y=w265) -> (x < y?=w270:bool)
            n163 = Select(t=DigitizerState."GetData", s=w270, f=DigitizerState."SendtoHost") -> (s? t:f=w268:T2)
            n164 = case shown="False" w270 {
              tunnel: [u16 0 ("Sample Count") w283] -> w266
              tunnel: w269 -> [_ w283]
              frame False {
              }
              frame True {
              }
            }
          }
          frame "SendtoHost" {
            n165 = xnode ("FIFO Method Node")("Timeout"=0) -> ("Element"=w354:u64, "Timed Out?"=w345:bool)  [unwired: 1 in, 1 out]
            n166 = case shown="False" w345 {
              tunnel: w354 -> [w357 _]
              frame False {
                n167 = xnode ("FIFO Method Node")("Element"=w357, "Timeout"=0) -> ("Timed Out?"=w359:bool)  [unwired: 1 in, 1 out]
                n168 = feedback #16(FALSE) -> (w360:bool)
                n169 = Compound Arithmetic op=OR(w360, w359) -> (w358:bool)
                "DMA FIFO Overflow? 2" <- w358
                n170 = feedback-in #16(w358) -> ()
              }
              frame True {
              }
            }
            n171 = Increment(x=w349) -> (x+1=w350:u16)
            n172 = Less?(x=w350, y=w348) -> (x < y?=w347:bool)
            n173 = case shown="False" w347 {
              tunnel: [u16 0 ("Sample Count") w364] -> w346
              tunnel: w350 -> [_ w364]
              frame False {
              }
              frame True {
              }
            }
            n174 = Select(t=DigitizerState."SendtoHost", s=w347, f=DigitizerState."Init") -> (s? t:f=w351:T2)
          }
        }
        "Data Transfer Loop" <- w213
      }
      n175 = node-c288(w203) -> ()
    }
    frame Disabled {
    }
  }
  n176 = node-c288() -> (w9:T4)  [unwired: 1 in]
  n177 = timed-loop "Analog Input" {
    timing: w9 -> [_]
    timing-out: [_] -> w8
    shift-right: [w403] -> _
    shift-left: Aquire_State."Idle" ("Acquire State") -> [w393]
    shift-right: [w404] -> _
    shift-left: w6 -> [w394]
    shift-right: [w402] -> _
    shift-left: w5 -> [w392]
    shift-right: [w379] -> _
    shift-left: _ -> [w378]
    shift-right: [w377] -> _
    shift-left: _ -> [w376]
    shift-right: [w374] -> _
    shift-left: w2 -> [w375]
    shift-right: [w372] -> _
    shift-left: w1 -> [w371]
    stop <- _ stop-if-true
    n178 = xnode "FPGA I/O Node"() -> ("IO Module\\AI 1 Data N-3"=w385:i16, "IO Module\\AI 0 Data N-3"=w384:i16, "IO Module\\AI 1 Data N-2"=w383:i16, "IO Module\\AI 0 Data N-2"=w382:i16, "IO Module\\AI 1 Data N-1"=w386:i16, "IO Module\\AI 0 Data N-1"=w387:i16, "IO Module\\AI 1 Data N"=w388:i16, "IO Module\\AI 0 Data N"=w389:i16)  [unwired: 8 in, 8 out]
    n179 = xnode ("FIFO Method Node")("Timeout"=0) -> ("Element"=w380:bool)  [unwired: 1 in, 2 out]
    n180 = Join Numbers(hi=w385, lo=w384) -> ((hi.lo)=w397:u32)
    n181 = Join Numbers(hi=w383, lo=w382) -> ((hi.lo)=w399:u32)
    n182 = Join Numbers(hi=w386, lo=w387) -> ((hi.lo)=w398:u32)
    n183 = Join Numbers(hi=w388, lo=w389) -> ((hi.lo)=w400:u32)
    n184 = Join Numbers(hi=w398, lo=w400) -> ((hi.lo)=w390:u64)
    n185 = Join Numbers(hi=w397, lo=w399) -> ((hi.lo)=w391:u64)
    n186 = feedback-in #17(w380) -> ()
    n187 = feedback #17() -> (w373:bool)  [unwired: 1 in]
    n188 = Bundle By Name(cluster=cluster{"Older Data":u64, "Newer Data":u64} {"Older Data"=0, "Newer Data"=0} ("Element"), "Older Data"=w391, "Newer Data"=w390) -> (w395:cluster{"Older Data":u64, "Newer Data":u64})
    n189 = feedback #18() -> (w401:cluster{"Older Data":u64, "Newer Data":u64})  [unwired: 1 in]
    n190 = feedback-in #18(w395) -> ()
    n191 = case shown="\"Acquire\"" w393 {
      tunnel: [u16 0 u16 0 w457 w469 w478 w500 u16 0] -> w404
      tunnel: w394 -> [_ _ w457 w468 w493 w502 _]
      tunnel: [w416 w428 w460 w472 w492 w505 w516] -> w403
      tunnel: [w413 w432 w458 w470 w489 w503 w514] -> w402
      tunnel: w392 -> [_ w432 w458 w470 w489 w503 w514]
      tunnel: w401 -> [_ w431 _ _ w488 _ _]
      tunnel: w373 -> [_ w426 _ _ _ _ _]
      tunnel: [w411 w424 w456 w467 w482 w501 w513] -> w379
      tunnel: w378 -> [_ w424 w456 w467 w482 w501 w513]
      tunnel: [w409 w423 w455 w465 w481 w498 w511] -> w377
      tunnel: w376 -> [_ w423 w455 w465 w481 w498 w511]
      tunnel: [u16 0 ("Avg Count") w422 w454 w464 w480 w497 w510] -> w374
      tunnel: w375 -> [_ w422 w454 w464 w480 w497 w512]
      tunnel: [w405 w420 w452 w462 w476 w496 w507] -> w372
      tunnel: w371 -> [_ w420 w452 w462 w476 w496 w507]
      frame "Idle", Default {
        # "This state will wait for the host VI to arm the trigger."
        n192 = feedback-in #19("Arm Trigger") -> ()
        n193 = feedback #19() -> (w414:bool)  [unwired: 1 in]
        n194 = local read "WaitForWave\nCompletion"() -> (w406:u16)
        n195 = Select(t=Aquire_State."Wait for Trigger" ("Acquire State"), s=w414, f=Aquire_State."Idle" ("Acquire State")) -> (s? t:f=w416:T1)
        n196 = local read "Delay after Trig [cycles]"() -> (w412:u16)
        n197 = local read "AvgCount"() -> (w410:u16)
        n198 = local read "Samples Per Trigger"() -> (w407:u16)
        n199 = feedback #20() -> (w411:u16)  [unwired: 1 in]
        n200 = feedback-in #20(w412) -> ()
        n201 = feedback #21() -> (w409:u16)  [unwired: 1 in]
        n202 = feedback-in #21(w410) -> ()
        n203 = feedback #22() -> (w405:u16)  [unwired: 1 in]
        n204 = feedback-in #22(w406) -> ()
        n205 = feedback-in #23(w407) -> ()
        n206 = feedback #23() -> (w413:u16)  [unwired: 1 in]
      }
      frame "Wait for Trigger" {
        # "After the trigger is armed, this state monitors for the specific trigger condition to begin the acquisition."
        n207 = feedback-in #24("Trigger Type") -> ()
        n208 = feedback #24() -> (w425:T3)  [unwired: 1 in]
        n209 = case shown="\"Software\", Default" w425 {
          tunnel: w431 -> [_ w451]
          tunnel: [w442 w443] -> w421
          tunnel: w426 -> [w437 _]
          frame "Software", Default {
            n210 = Compound Arithmetic op=AND(w437, invert "vi/nGenTrig") -> (w441:bool)
            n211 = Compound Arithmetic op=AND("vi/nGenTrig", "TrigIn Simulate") -> (w439:bool)
            n212 = Compound Arithmetic op=OR(w441, w439) -> (w436:bool)
            n213 = call <instrlib>:"Detect Rising Edge.vi"("signal"=w436) -> ("edge detected"=w442:bool)  [unwired: 14 in]
          }
          frame "Data Edge" {
            # "Begins the acquisition after the analog input rises above the trigger level."
            n214 = Unbundle By Name(w451) -> ("Older Data"=w449:u64, "Newer Data"=w447:u64)
            n215 = feedback-in #25("Trigger Level") -> ()
            n216 = feedback #25() -> (w445:i16)  [unwired: 1 in]
            n217 = feedback-in #26(w449) -> ()
            n218 = feedback #26() -> (w444:u64)  [unwired: 1 in]
            n219 = feedback-in #27(w447) -> ()
            n220 = feedback #27() -> (w446:u64)  [unwired: 1 in]
            n221 = call "Data Edge Trigger 8 Samples.vi"("Trigger Level"=w445, "Newer Data In"=w446, "Older Data In"=w444) -> ("Trigger"=w450:bool)  [unwired: 8 in]
            n222 = feedback-in #28(w450) -> ()
            n223 = feedback #28() -> (w443:bool)  [unwired: 1 in]
          }
        }
        n224 = case shown="True" w421 {
          selector: w421 -> [_ w435]
          frame False {
          }
          frame True {
            n225 = xnode ("FIFO Method Node")("Element"=w435, "Timeout"=0) -> ()  [unwired: 1 in, 2 out]
          }
        }
        n226 = Select(t=Aquire_State."AlignWave" ("Acquire State"), s=w421, f=Aquire_State."Wait for Trigger") -> (s? t:f=w428:T1)
      }
      frame "AlignWave" {
        n227 = xnode "FPGA I/O Node"() -> ("PXI_Trig0"=w453:bool)  [unwired: 1 in, 1 out]
        n228 = Select(t=Aquire_State."Hold Aquire" ("Acquire State"), s=w453, f=Aquire_State."AlignWave" ("Acquire State")) -> (s? t:f=w460:T1)
      }
      frame "Hold Aquire" {
        n229 = Increment(x=w468) -> (x+1=w466:u16)
        n230 = Greater?(x=w467, y=w466) -> (0:w463:bool)
        n231 = Select(t=Aquire_State."Hold Aquire" ("Acquire State"), s=w463, f=Aquire_State."Acquire" ("Acquire State")) -> (s? t:f=w472:T1)
        n232 = case shown="True" w463 {
          tunnel: [u16 0 w475] -> w469
          tunnel: w466 -> [_ w475]
          frame False {
          }
          frame True {
          }
        }
      }
      frame "Acquire" {
        # "Monitor for any  FIFO timeouts"
        # "While in this state, data is pushed into a DMA FIFO until the desired number of samples per record have been acquired."
        n233 = xnode ("FIFO Method Node")("Element"=w488, "Timeout"=0) -> ("Timed Out?"=w483:bool)  [unwired: 1 in, 1 out]
        n234 = Increment(x=w493) -> (x+1=w479:u16)
        n235 = Less?(x=w479, y=w489) -> (x < y?=w477:bool)
        n236 = feedback #29(FALSE) -> (w484:bool)
        n237 = Or(x=w484, y=w483) -> (x .or. y?=w485:bool)
        "TS FIFO In Overflow?" <- w485
        n238 = feedback-in #29(w485) -> ()
        n239 = Select(t=Aquire_State."Acquire" ("Acquire State"), s=w477, f=Aquire_State."WaitForWaveCompletion" ("Acquire State")) -> (s? t:f=w492:T1)
        n240 = case shown="False" w477 {
          tunnel: w479 -> [_ w495]
          tunnel: [u16 0 w495] -> w478
          frame False {
          }
          frame True {
          }
        }
      }
      frame "WaitForWaveCompletion" {
        n241 = Increment(x=w502) -> (x+1=w500:u16)
        n242 = Greater?(x=w496, y=w500) -> (0:w499:bool)
        n243 = Select(t=Aquire_State."WaitForWaveCompletion" ("Acquire State"), s=w499, f=Aquire_State."CheckAvg" ("Acquire State")) -> (s? t:f=w505:T1)
      }
      frame "CheckAvg" {
        n244 = Increment(x=w512) -> (x+1=w510:u16)
        n245 = Greater?(x=w511, y=w510) -> (0:w508:bool)
        n246 = Select(t=Aquire_State."AlignWave" ("Acquire State"), s=w508, f=Aquire_State."Idle") -> (s? t:f=w516:T1)
        n247 = xnode ("FIFO Method Node")("Element"=w508, "Timeout"=0) -> ()  [unwired: 1 in, 2 out]
      }
    }
    "Aquire Loop" <- w393
  }
  n248 = while "Configuration Loop" {
    stop <- FALSE stop-if-true
    # "After the NI 5772 is powered on, the CLIP core provides the module with a default configuration. This loop updates the host VI to the status of the NI 5772 through the Initalization Done Signal. Additionally, this loop configures the Sample clock selection for the NI 5772. Refer to the Clock Select (Host).vi Host VI for more information about how this example configures the clock."
    n249 = xnode "FPGA I/O Node"("IO Module\\User Command"="User Command", "IO Module\\User Data 0"="User Data 0", "IO Module\\User Data 1"="User Data 1", "IO Module\\User Command Commit"="User Command Commit") -> ("IO Module\\User Command Idle"=→"User Command Idle":bool, "IO Module\\User Command Status"=→"User Command Status":u8, "IO Module\\PLL Locked"=→"PLL Locked":bool, "IO Module\\User Error"=w526:u8, "IO Module\\Initialization Done"=→"Configured?":bool)  [unwired: 9 in, 9 out]
    n250 = Not Equal To 0?(x=w526) -> (x != 0?=→"User Error":bool)
  }
  n251 = while "Data Validation/Calculation Loop" {
    stop <- FALSE stop-if-true
    n252 = Scale By Power Of 2(n="AvgCount_powerOf2", x=1 ("Timeout")) -> (x*2^n=w552:i32)
    n253 = To Unsigned Word Integer(number=w552) -> (unsigned 16bit integer=w549:u16)
    n254 = Multiply(x="Delay (us)", y=sgl 200.0) -> (x*y=w545:u16)
    n255 = Divide(x="WaveSampleCount", y="Wave Sampling Rate") -> (x/y=w537:sgl)
    n256 = In Range and Coerce(upper limit=u16 65535, x=w545, lower limit=u16 1) -> (coerced(x)=w538:u16)  [unwired: 1 out]
    "Delay after Trig [cycles]" <- w538
    n257 = In Range and Coerce(upper limit=u16 65535, x=w549, lower limit=u16 1) -> (coerced(x)=→"AvgCount":u16)  [unwired: 1 out]
    n258 = Multiply(x=w537, y=sgl 200000000.0) -> (x*y=w534:sgl)
    n259 = Add(x="Samples Per Trigger", y=w538) -> (x+y=w535:u16)
    n260 = Subtract(x=w534, y=w535) -> (x-y=→"WaitForWave\nCompletion":u16)
    n261 = call "Loop Timer"("Count(uSec)"=u32 100 ("Count(mSec)")) -> ()  [unwired: 1 out]
  }
  n262 = while "TrigOut Loop" {
    stop <- FALSE stop-if-true
    n263 = xnode ("FIFO Method Node")("Timeout"=0) -> ("Element"=w555:bool)  [unwired: 1 in, 2 out]
    n264 = case shown="True" w555 {
      frame False {
      }
      frame True {
        n265 = flat-sequence {
          frame #0 {
            n266 = xnode "FPGA I/O Node"("PXI_Trig1"=TRUE) -> ()  [unwired: 1 in, 1 out]
          }
          frame #1 {
            n267 = call "Wait"("Count(Ticks)"=u32 20 ("Count(uSec)")) -> ()  [unwired: 1 out]
          }
          frame #2 {
            n268 = xnode "FPGA I/O Node"("PXI_Trig1"=FALSE) -> ()  [unwired: 1 in, 1 out]
          }
        }
      }
    }
  }
  n269 = node-c288() -> (w4:T4)  [unwired: 1 in]
  n270 = timed-loop "Trigger In Loop" {
    timing: w4 -> [_]
    timing-out: [_] -> w3
    stop <- FALSE stop-if-true
    # "Triggering is handeled in the 40MHz Loop to remove the signal Jitter and false triggers"
    n271 = xnode "FPGA I/O Node"() -> ("IO Module\\Asynchronous Trigger Input"=w566:bool)  [unwired: 1 in, 1 out]
    n272 = call <instrlib>:"Detect Rising Edge.vi"("signal"=w566) -> ("edge detected"=w563:bool)  [unwired: 14 in]
    n273 = xnode ("FIFO Method Node")("Element"=w566, "Timeout"=0) -> ()  [unwired: 1 in, 2 out]
    n274 = call-poly <instrlib>:"Count Up.vi"("increment"=w563, "reset"="Clear Count") -> ("count out"=→"Trig Count":u64)  [unwired: 13 in]
  }
  n275 = node-c288(w3) -> ()
  n276 = node-c288(w8) -> ()
